vi "spec_GetCenterWavelength.vi"(8 "error in (no error)":errorcluster, 11 "LightField Automation in":refnum<class "LightField Automation.lvclass">) -> (0 "error out":errorcluster, 2 "Center Wavelenght":dbl, 3 "LightField Automation out":refnum<class "LightField Automation.lvclass">)   [LabVIEW 2013, in "LightField Automation.lvclass"]
uses:
  LightField Automation.lvclass
  C:/Program Files/Princeton Instruments/LightField/PrincetonInstruments.LightFieldAddInSupportServices.dll
  Program Files/Princeton Instruments/LightField/PrincetonInstruments.LightFieldAddInSupportServices.dll
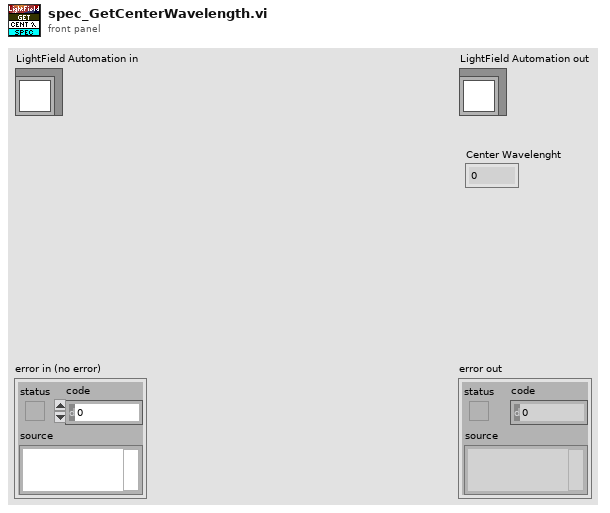
[diagram p1: front panel]
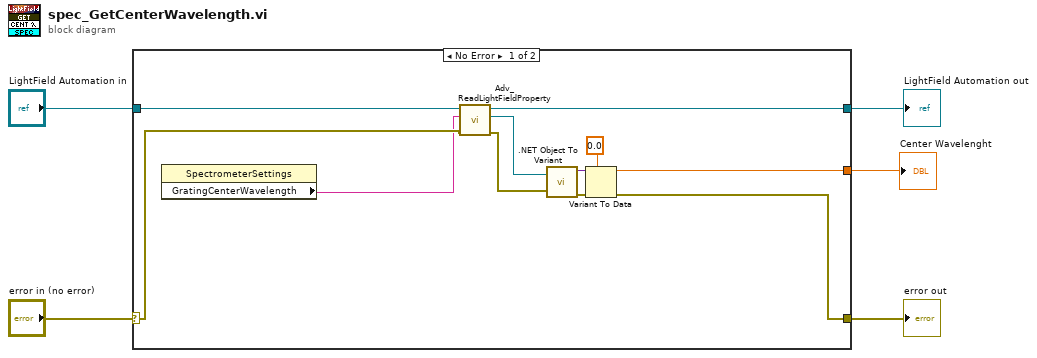
[diagram p0: block diagram]
diagram:
  n1 = case shown="No Error" "error in (no error)" {
    selector: "error in (no error)" -> [w8 w18]
    tunnel: [w6 w18] -> w4
    tunnel: [w11 w17] -> w2
    tunnel: "LightField Automation in" -> [w9 w17]
    tunnel: [w10 _] -> w1
    frame No Error {
      n2 = property class="SpectrometerSettings"() -> ("GratingCenterWavelength"=w7:string)  [unwired: 2 in, 2 out]
      n3 = call "Adv_ReadLightFieldProperty.vi"("error in (no error)"=w8, "setting"=w7, "LightField Automation in"=w9) -> ("error out"=w15:errorcluster, "value"=w16:refnum<k24>, "LightField Automation out"=w11:refnum<class "LightField Automation.lvclass">)  [unwired: 6 in]
      n4 = call <vilib>:".NET Object To Variant.vi"("error in (no error)"=w15, ".NET object"=w16) -> ("error out"=w12:errorcluster, "variant"=w14:variant)
      n5 = Variant To Data(error in=w12, type=0.0, Variant=w14) -> (data=w10:dbl, error out=w6:errorcluster)
    }
    frame Error {
    }
  }
  "error out" <- w4
  "LightField Automation out" <- w2
  "Center Wavelenght" <- w1
